vi "AH2500_singel_read_visa.vi"(0 "VISA-AH2500-address":refnum<visa-resource-name>, 2 "error in (no error)":errorcluster caption="Fehler (Eingang, kein Fehler)") -> (3 "Capacity":dbl, 4 "Loss":dbl, 6 "error out":errorcluster caption="Fehler (Ausgang)")   [LabVIEW 2019]
uses:
  Instrument_Setup.vi
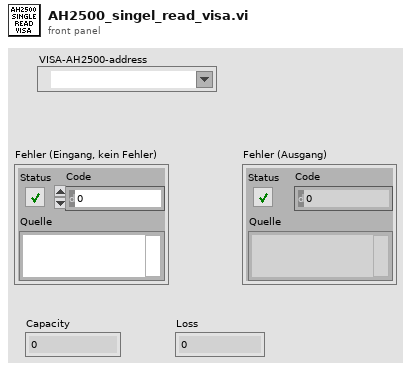
[diagram p1: front panel]
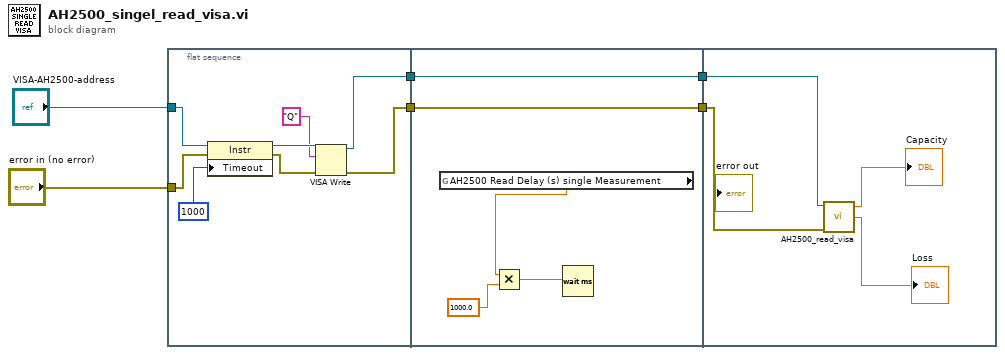
[diagram p0: block diagram]
diagram:
  n1 = flat-sequence {
    tunnel: "VISA-AH2500-address" -> [w14]
    tunnel: "error in (no error)" -> [w13]
    tunnel: [w8] -> w3
    tunnel: [w7] -> w2
    tunnel: [w16] -> w4
    tunnel: w3 -> [w16]
    tunnel: w2 -> [w15]
    tunnel: [w15] -> w1
    tunnel: w4 -> [w23]
    tunnel: w1 -> [w22]
    frame #0 {
      n2 = property class="Instr"(reference=w14, error in=w13, "Timeout"=1000) -> (reference out=w11:refnum<visa-resource-name>, error out=w10:errorcluster)
      n3 = VISA Write(VISA resource name=w11, write buffer="Q", error in (no error)=w10) -> (VISA resource name out=w8:refnum<visa-resource-name>, error out=w7:errorcluster)  [unwired: 1 out]
    }
    frame #1 {
      n4 = global read "Instrument_Setup.vi" "AH2500 Read Delay (s) single Measurement"() -> (w18:dbl)
      n5 = Multiply(x=w18, y=1000.0) -> (x*y=w19:dbl)
      n6 = Wait (ms)(milliseconds to wait=w19) -> ()  [unwired: 1 out]
    }
    frame #2 {
      n7 = call "AH2500_read_visa.vi"("error in (no error)"=w22, "VISA-AH2500A-address"=w23) -> ("loss"=→"Loss":dbl, "capacitance"=→"Capacity":dbl)  [unwired: 2 in, 1 out]
    }
  }
